vi "ManipChangePiece.vi"(3 "Parameter String":string) -> (0 "error out":errorcluster, 1 "Advance Trigger":bool)   [LabVIEW 2020]
doc: "This VI changes what game peice you're using in auto.\n\nParameters:\nDecides what game peice you use (\"cube\" or \"cone\")"
uses:
  SafeParser_String.vi
  GlobalDriverStationCommands.vi
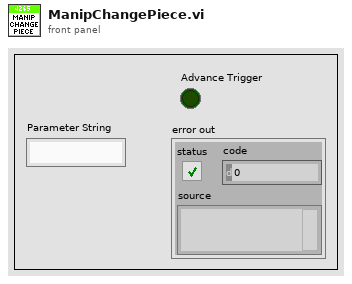
[diagram p1: front panel]
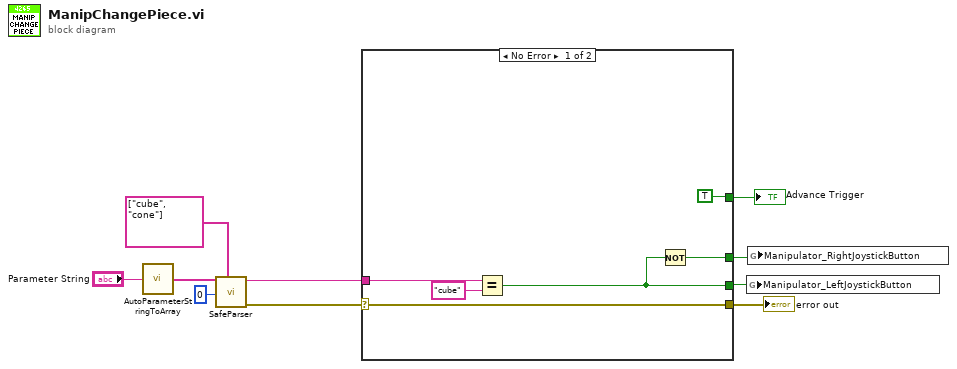
[diagram p0: block diagram]
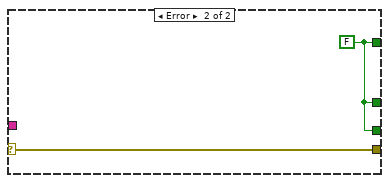
[diagram p2: hidden frame]
diagram:
  n1 = call "AutoParameterStringToArray.vi"("Parameter String"="Parameter String") -> ("Parsed Parameters"=w8:string[])
  n2 = call-poly "SafeParser.vi"("Allowed Values"=string[] ["cube", "cone"], "Array Index"=0 ("Parameter Index"), "String Array"=w8) -> ("Error Out"=w6:errorcluster, "Typecast Value"=w4:string)  [unwired: 7 in]
  n3 = case shown="No Error" w6 {
    selector: w6 -> [w16 w18]
    tunnel: [w12 w17] -> w2
    tunnel: [w16 w18] -> w5
    tunnel: w4 -> [w15 _]
    tunnel: [TRUE w17] -> w3
    tunnel: [w11 w17] -> w1
    frame No Error {
      n4 = Equal?(x=w15, y="cube") -> (x = y?=w12:bool)
      n5 = Not(x=w12) -> (.not. x?=w11:bool)
    }
    frame Error {
      w17 = FALSE
    }
  }
  "Advance Trigger" <- w3
  "error out" <- w5
  n6 = global write "GlobalDriverStationCommands.vi" "Manipulator_LeftJoystickButton"(w2) -> ()
  n7 = global write "GlobalDriverStationCommands.vi" "Manipulator_RightJoystickButton"(w1) -> ()
